vi "Get Source Status Info from RunSet.vi"(10 "Tags":T1[](array[typedef]), 11 "Source":refnum<class "Source.lvclass">) -> (3 "Tag Status Info":T2[](array[typedef]))   [LabVIEW 2013, in "Customer.TestSLATE.Mnemonic.lvlib"]
doc: "Loads channel status info into array of clusters in this order:\n0 AI\n1 AO\n2 FI\n3 CA\n4 DO\n5 DI"
uses:
  Customer.TestSLATE.Mnemonic.lvlib
  Source Status Information.ctl
  <vilib>/Test SLATE/CVT/Tag Information.ctl
  <vilib>/Test SLATE/CLASSES/TAG/TS_Tag.lvclass
  <vilib>/Test SLATE/CLASSES/SOURCE/Source.lvclass
  <vilib>/Test SLATE/Test SLATE.lvlib
panel:
  # "`"
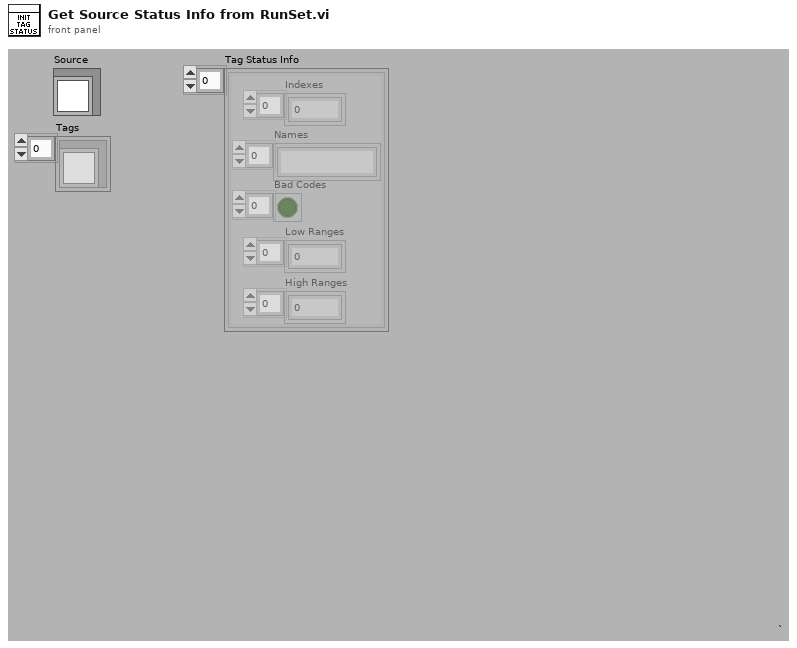
[diagram p1: front panel]
types:
  T1 = typedef "Test SLATE.lvlib/Tag Information.ctl" = refnum<class "TS_Tag.lvclass">
  T2 = typedef "Customer.TestSLATE.Mnemonic.lvlib/Source Status Information.ctl" = cluster{"Indexes":i32[], "Names":string[], "Bad Codes":bool[], "Low Ranges":sgl[], "High Ranges":sgl[]}
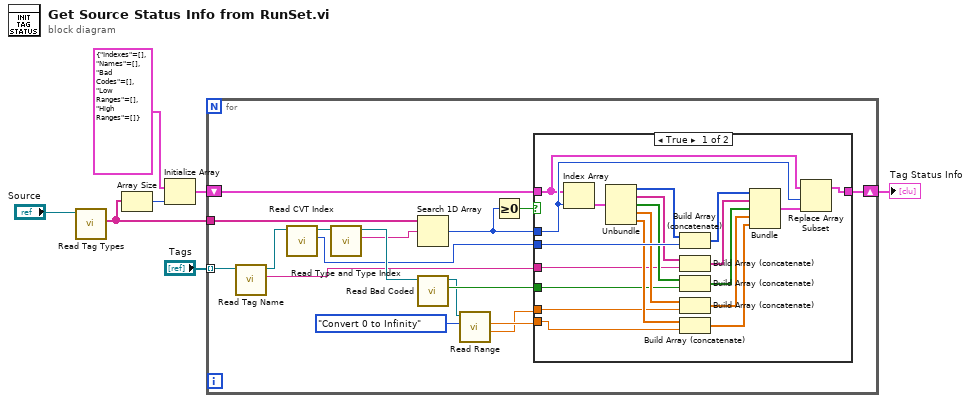
[diagram p0: block diagram]
diagram:
  n1 = call <vilib>:"Read Tag Types.vi"("Source in"="Source") -> ("Tag Types"=w2:string[])  [unwired: 9 in, 1 out]
  n2 = Array Size(array=w2) -> (size(s)=w4:i32)
  n3 = Initialize Array(T2 {"Indexes"=[], "Names"=[], "Bad Codes"=[], "Low Ranges"=[], "High Ranges"=[]} ("Status Info"), w4) -> (w3:T2[])
  n4 = for {
    tunnel: "Tags" -> [w15] mode=indexing
    shift-right: [w8] -> w1
    shift-left: w3 -> [w10]
    tunnel: w2 -> [w12]
    n5 = call <vilib>:"Read Tag Name.vi"("Tag in"=w15) -> ("Tag Name"=w14:string, "Tag out"=w16:T1)  [unwired: 9 in]
    n6 = call <vilib>:"Read CVT Index.vi"("Tag in"=w16) -> ("CVT Index"=w17:i32, "Tag out"=w18:T1)  [unwired: 9 in]
    n7 = call <vilib>:"Read Type and Type Index.vi"("Tag in"=w18) -> ("Type"=w13:string, "Tag out"=w24:T1)  [unwired: 8 in, 1 out]
    n8 = Search 1D Array(1D array=w12, element=w13) -> (index of element=w9:i32)  [unwired: 1 in]
    n9 = call <vilib>:"Read Bad Coded.vi"("Tag in"=w24) -> ("Bad Coded?"=w23:bool, "Tag out"=w22:T1)  [unwired: 9 in]
    n10 = call <vilib>:"Read Range.vi"("Reset"=enum16{"No Change", "Convert 0 to Infinity"}."Convert 0 to Infinity", "Tag in"=w22) -> ("Range.Low"=w19:dbl, "Range.High"=w20:dbl)  [unwired: 7 in, 1 out]
    n11 = Greater Or Equal To 0?(x=w9) -> (x >= 0?=w11:bool)
    n12 = case shown="True" w11 {
      tunnel: w23 -> [w36 _]
      tunnel: w19 -> [w37 _]
      tunnel: w20 -> [w38 _]
      tunnel: w14 -> [w35 _]
      tunnel: w17 -> [w43 _]
      tunnel: [w25 w45] -> w8
      tunnel: w10 -> [w26 w45]
      tunnel: w9 -> [w28 _]
      frame True {
        n13 = Index Array(array=w26, index=w28) -> (element=w29:T2)
        n14 = Unbundle(w29) -> ("Indexes"=w44:i32[], "Names"=w42:string[], "Bad Codes"=w41:bool[], "Low Ranges"=w40:sgl[], "High Ranges"=w39:sgl[])
        n15 = Build Array (concatenate)(w44, w43) -> (w34:i32[])
        n16 = Build Array (concatenate)(w42, w35) -> (w33:string[])
        n17 = Build Array (concatenate)(w41, w36) -> (w32:bool[])
        n18 = Build Array (concatenate)(w40, w37) -> (w31:dbl[])
        n19 = Build Array (concatenate)(w39, w38) -> (w30:dbl[])
        n20 = Bundle(w34, w33, w32, w31, w30) -> (w27:cluster{i32[], string[], bool[], dbl[], dbl[]})  [unwired: 1 in]
        n21 = Replace Array Subset(array=w26, new element=w27, index=w28) -> (w25:T2[])
      }
      frame False {
      }
    }
  }
  "Tag Status Info" <- w1
